vi "Add Pattern.vi"(6 "Advanced Options":cluster{"Item":u16, "Value":dbl}[](array[cluster]) {"Item" items=["LD Sampling - Search Strategy Support"=0, "LD Sampling - Initial Step Size"=1, "LD Sampling - Initial Sample Size"=2, "LD Sampling - Initial Sample Size Factor"=3, "LD Sampling - Initial Angular Accuracy"=4, "LD Sampling - Final Sample Size"=5, "LD Sampling - Final Sample Size Factor"=6, "LD Sampling - Final Angular Accuracy"=7, "LD Sampling - Subpixel Sample Size"=8, "LD Sampling - Subpixel Sample Size Factor"=9, "LD Sampling - Match Offset X Position"=10, "LD Sampling - Match Offset Y Position"=11, "LD Sampling - Match Offset Angle"=12, "-"=13, "Pyramid - Subpixel Sample Size"=100, "Pyramid - Subpixel Sample Size Factor"=101, "Pyramid - Match Offset X Position"=102, "Pyramid - Match Offset Y Position"=103, "Pyramid - Match Offset Angle"=104, "Pyramid - Max Pyramid Level To Store Data"=105]}, 7 "Save to Library?":bool, 8 "error in (no error)":errorcluster, 9 "Image Name":string, 10 "Image":T1, 11 "MultiPattern Matcher in":refnum<class "MultiPattern Matcher.lvclass">) -> (0 "error out":errorcluster, 3 "MultiPattern Matcher out":refnum<class "MultiPattern Matcher.lvclass">)   [LabVIEW 2013, in "MultiPattern Matcher.lvclass"]
uses:
  MultiPattern Matcher.lvclass
  <vilib>/vision/Image Controls.llb/IMAQ Image.ctl
  MultiPattern Matcher.lvclass/MultiPattern Matcher.ctl
  <vilib>/vision/NI_Vision_Development_Module.lvlib
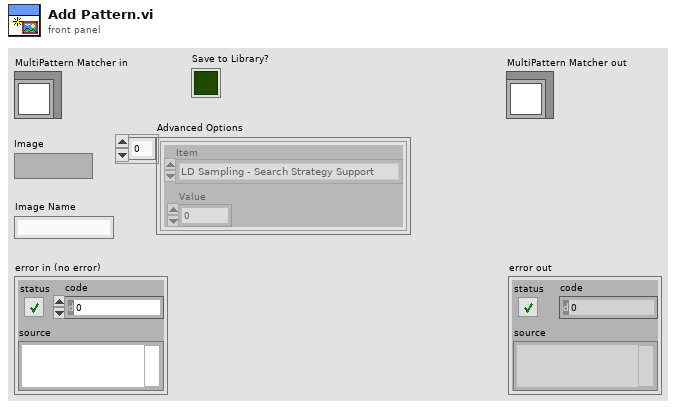
[diagram p1: front panel]
types:
  T1 = typedef "IMAQ Image.ctl" = refnum<image>
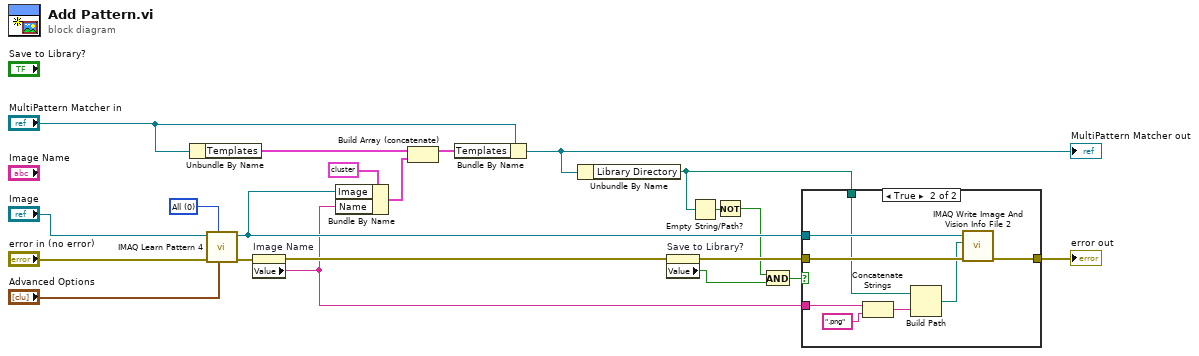
[diagram p0: block diagram]
diagram:
  w19 = 0 items=["All", "Low Discrepancy Sampling", "Grayscale Value Pyramid", "Gradients Pyramid"] ("Algorithm")
  n1 = Unbundle By Name("MultiPattern Matcher in") -> ("Templates"=w15:cluster{"Image":T1, "Name":string}[])
  n2 = call "IMAQ Learn Pattern 4"("Advanced Options"="Advanced Options", "Algorithm"=w19, "error in (no error)"="error in (no error)", "Image"="Image") -> ("error out"=w17:errorcluster, "Template Image Out"=w10:T1)  [unwired: 5 in, 1 out]
  n3 = property on="Image Name" class="Str"(error in=w17) -> (error out=w12:errorcluster, "Value"=w8:string)  [unwired: 1 in, 1 out]
  n4 = Bundle By Name(cluster=cluster{"Image":T1, "Name":string} {"Image"=refnum, "Name"=""} ("Cluster"), "Image"=w10, "Name"=w8) -> (w13:cluster{"Image":T1, "Name":string})
  n5 = Build Array (concatenate)(w15, w13) -> (w14:cluster{"Image":T1, "Name":string}[])
  n6 = Bundle By Name(cluster="MultiPattern Matcher in", "Templates"=w14) -> (w7:refnum<class "MultiPattern Matcher.lvclass">)
  "MultiPattern Matcher out" <- w7
  n7 = Unbundle By Name(w7) -> ("Library Directory"=w6:path)
  n8 = property on="Save to Library?" class="Bool (strict)"(error in=w12) -> (error out=w11:errorcluster, "Value"=w3:bool)  [unwired: 1 in, 1 out]
  n9 = Empty String/Path?(string/path=w6) -> (empty?=w5:bool)
  n10 = Not(x=w5) -> (.not. x?=w2:bool)
  n11 = And(x=w2, y=w3) -> (x .and. y?=w4:bool)
  n12 = case shown="True" w4 {
    tunnel: w11 -> [w22 w30]
    tunnel: [w22 w28] -> w9
    tunnel: w10 -> [_ w29]
    tunnel: w8 -> [_ w24]
    tunnel: w6 -> [_ w23]
    frame False {
    }
    frame True {
      n13 = Concatenate Strings(w24, ".png" ("string")) -> (w27:string)
      n14 = Build Path(base path=w23, name or relative path=w27) -> (appended path=w26:path)
      n15 = call "IMAQ Write Image And Vision Info File 2"("error in (no error)"=w30, "File Path"=w26, "Image"=w29) -> ("error out"=w28:errorcluster)  [unwired: 7 in, 1 out]
    }
  }
  "error out" <- w9
